vi "GetScaleList.vi"(10 "Data in":T1, 11 "Bitfield in":string) -> (3 "output array":string[](array[string]))   [LabVIEW 2017]
uses:
  Ctrl/Property.ctl
  Ctrl/PhysicalChannel.ctl
  Ctrl/Bitfield.ctl
  Ctrl/Register.ctl
  Ctrl/ScaleType.ctl
  Ctrl/Scale.ctl
  Ctrl/EnumValue.ctl
  Ctrl/Enum.ctl
  Ctrl/Caps.ctl
  Ctrl/Data.ctl
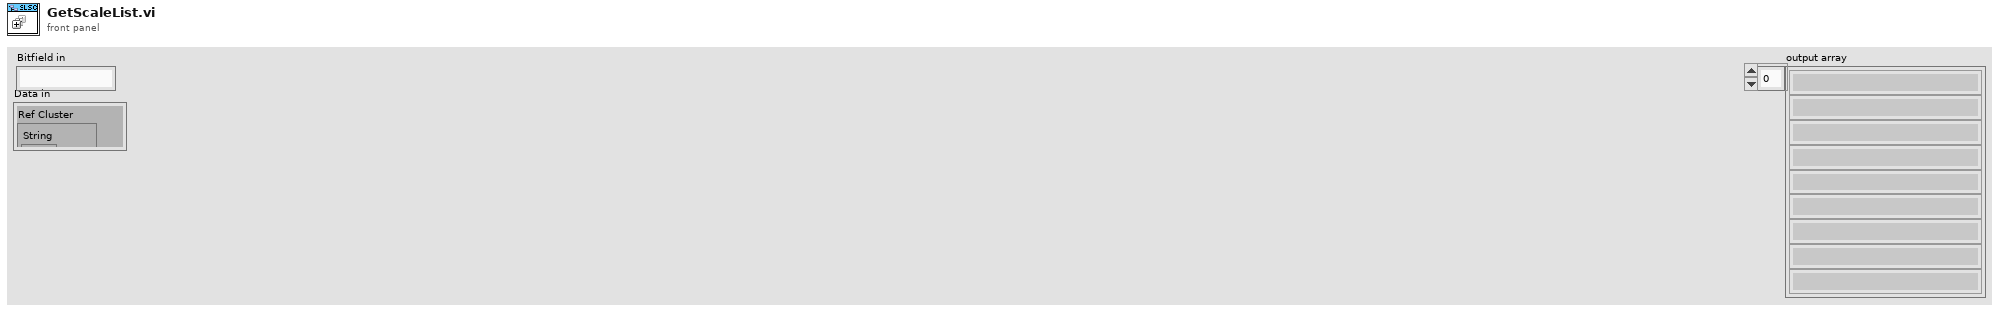
[diagram p1: front panel]
types:
  T1 = typedef "Data.ctl" = cluster{"Ref Cluster":cluster{"String":refnum<vi>, "U8":refnum<vi>, "I8":refnum<vi>, "U32":refnum<vi>, "I32":refnum<vi>, "U64":refnum<vi>, "I64":refnum<vi>, "Ring":refnum<vi>, "DBL":refnum<vi>, "Add":refnum<vi>, "Remove":refnum<vi>, "Property tree":refnum<vi>, "confirm":refnum<vi>}, "JSON Text":string, "Original JSON Text":string, "Caps":T2, "SLSC Output Tree":cluster{"Left Cell String":string, "Child Text":string[], "Child Tag":string, "Item Indent":i32, "Child Only?":bool, "Glyph Index":i32, "offline value":variant}[], "Ref Index and Control Type":cluster{"index":i32, "Datatype":string}, "Selected Type and name":cluster{"Selected Type":enum16{"Property", "Physical Channel", "Other"}, "Selected Property Name":string}, "Update whole Tree?":bool}
  T2 = typedef "Caps.ctl" = cluster{"properties":T3[], "physical channels":T4[], "registers":T5[], "scales":T7[], "enums":T9[], "productName":string}
  T3 = typedef "Property.ctl" = cluster{"name":string, "bitfield":string, "value":variant, "dataType":string, "min":variant, "max":variant, "scale":string, "access":string}
  T4 = typedef "PhysicalChannel.ctl" = cluster{"name":string, "properties":T3[]}
  T5 = typedef "Register.ctl" = cluster{"name":string, "address":i32, "size":i32, "bitfields":T6[], "initialValue":variant, "connectedProperties":string[]}
  T6 = typedef "Bitfield.ctl" = cluster{"name":string, "offset":i32, "size":i32, "signed":bool}
  T7 = typedef "Scale.ctl" = cluster{"name":string, "type":T8, "params":variant}
  T8 = typedef "ScaleType.ctl" = enum16{"NoScale", "Table", "Polynomial", "Linear"}
  T9 = typedef "Enum.ctl" = cluster{"name":string, "values":T10[]}
  T10 = typedef "EnumValue.ctl" = cluster{"name":string, "value":i32}
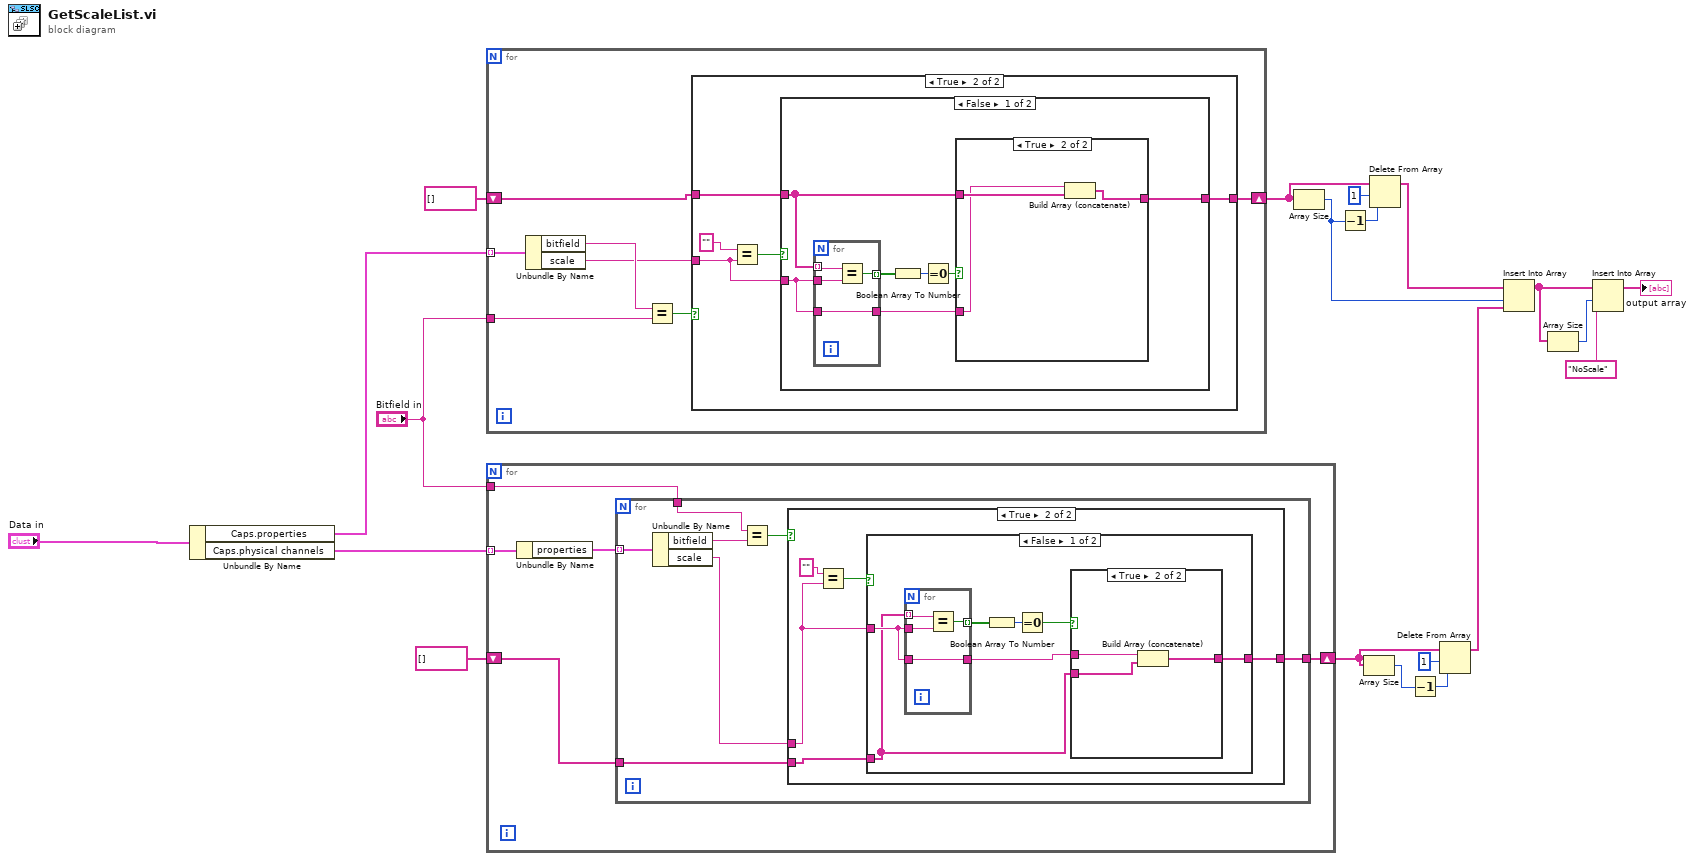
[diagram p0: block diagram]
diagram:
  n1 = Unbundle By Name("Data in") -> ("Caps.properties"=w6:T3[], "Caps.physical channels"=w5:T4[])
  n2 = for {
    tunnel: w6 -> [w27] mode=indexing
    tunnel: "Bitfield in" -> [w26]
    shift-right: [w21] -> w9
    shift-left: string[] [] -> [w23]
    n3 = Unbundle By Name(w27) -> ("bitfield"=w25:string, "scale"=w22:string)
    n4 = Equal?(x=w25, y=w26) -> (x = y?=w24:bool)
    n5 = case shown="True" w24 {
      tunnel: [w28 w33] -> w21
      tunnel: w23 -> [w28 w32]
      tunnel: w22 -> [_ w29]
      frame False {
      }
      frame True {
        n6 = Equal?(x="", y=w29) -> (x = y?=w30:bool)
        n7 = case shown="False" w30 {
          tunnel: [w34 w49] -> w33
          tunnel: w32 -> [w36 w49]
          tunnel: w29 -> [w37 _]
          frame False {
            n8 = for {
              tunnel: w36 -> [w48] mode=indexing
              tunnel: w37 -> [w47]
              tunnel: [w46] -> w40 mode=indexing
              tunnel: [w45] -> w35
              tunnel: w37 -> [w45]
              n9 = Equal?(x=w48, y=w47) -> (x = y?=w46:bool)
            }
            n10 = Boolean Array To Number(Boolean array=w40) -> (number=w39:u32)
            n11 = Equal To 0?(x=w39) -> (x = 0?=w38:bool)
            n12 = case shown="True" w38 {
              tunnel: w36 -> [w41 w43]
              tunnel: w35 -> [_ w42]
              tunnel: [w41 w44] -> w34
              frame False {
              }
              frame True {
                n13 = Build Array (concatenate)(w42, w43) -> (w44:string[])
              }
            }
          }
          frame True {
          }
        }
      }
    }
  }
  n14 = for {
    tunnel: w5 -> [w53] mode=indexing
    tunnel: "Bitfield in" -> [w52]
    shift-right: [w50] -> w15
    shift-left: string[] [] -> [w51]
    n15 = Unbundle By Name(w53) -> ("properties"=w54:T3[])
    n16 = for {
      tunnel: w54 -> [w61] mode=indexing
      tunnel: w52 -> [w59]
      tunnel: w51 -> [w57]
      tunnel: [w55] -> w50
      n17 = Unbundle By Name(w61) -> ("bitfield"=w60:string, "scale"=w56:string)
      n18 = Equal?(x=w59, y=w60) -> (x = y?=w58:bool)
      n19 = case shown="True" w58 {
        tunnel: w57 -> [w62 w67]
        tunnel: w56 -> [_ w64]
        tunnel: [w62 w63] -> w55
        frame False {
        }
        frame True {
          n20 = Equal?(x="", y=w64) -> (x = y?=w65:bool)
          n21 = case shown="False" w65 {
            tunnel: w67 -> [w70 w83]
            tunnel: w64 -> [w72 _]
            tunnel: [w68 w83] -> w63
            frame False {
              n22 = for {
                tunnel: w70 -> [w82] mode=indexing
                tunnel: w72 -> [w81]
                tunnel: [w80] -> w73 mode=indexing
                tunnel: [w79] -> w69
                tunnel: w72 -> [w79]
                n23 = Equal?(x=w82, y=w81) -> (x = y?=w80:bool)
              }
              n24 = Boolean Array To Number(Boolean array=w73) -> (number=w74:u32)
              n25 = Equal To 0?(x=w74) -> (x = 0?=w71:bool)
              n26 = case shown="True" w71 {
                tunnel: w70 -> [w75 w78]
                tunnel: w69 -> [_ w77]
                tunnel: [w75 w76] -> w68
                frame False {
                }
                frame True {
                  n27 = Build Array (concatenate)(w77, w78) -> (w76:string[])
                }
              }
            }
            frame True {
            }
          }
        }
      }
    }
  }
  n28 = Array Size(array=w9) -> (size(s)=w17:i32)
  n29 = Decrement(x=w17) -> (x-1=w11:i32)
  n30 = Array Size(array=w15) -> (size(s)=w13:i32)
  n31 = Delete From Array(array=w9, length=1, index=w11) -> (array with subset deleted=w16:string[])  [unwired: 1 out]
  n32 = Decrement(x=w13) -> (x-1=w12:i32)
  n33 = Delete From Array(array=w15, length=1, index=w12) -> (array with subset deleted=w18:string[])  [unwired: 1 out]
  n34 = Insert Into Array(array=w16, index=w17, new element=w18) -> (w4:string[])
  n35 = Array Size(array=w4) -> (size(s)=w3:i32)
  n36 = Insert Into Array(array=w4, index=w3, new element="NoScale" ("new element/subarray")) -> (→"output array":string[])
